vi "Read Tuner Type.vi"(8 "error in (no error)":errorcluster, 11 "RTL-SDR in":refnum<class "Session.lvclass">) -> (0 "error out":errorcluster, 3 "RTL-SDR out":refnum<class "Session.lvclass">)   [LabVIEW 2020, in "RTL-SDR.lvlib" / "Session.lvclass"]
uses:
  Session.lvclass
  Tuner Type.ctl
  RTL-SDR.lvlib
  C:/dev/IlluminatedG/lv-rtl-sdr/lib/librtlsdr.dll
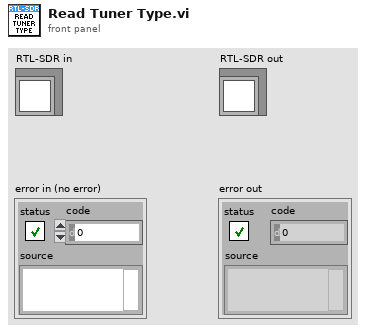
[diagram p1: front panel]
types:
  T1 = typedef "RTL-SDR.lvlib/Tuner Type.ctl" = enum32{"Unknown", "E4000", "FC0012", "FC0013", "FC2580", "R820T", "R828D"}
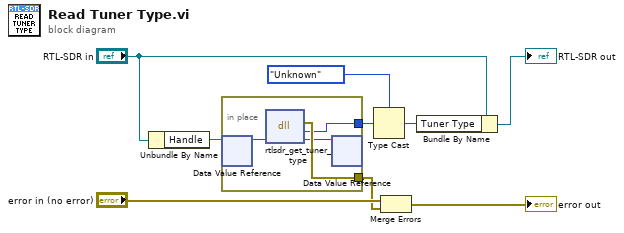
[diagram p0: block diagram]
diagram:
  n1 = Unbundle By Name("RTL-SDR in") -> ("Handle"=w1:refnum<data-value>)
  n2 = in-place {
    in-place-border: [w13] -> w6
    in-place-border: [w12] -> w5
    n3 = in-place-dvr #1(w1) -> (w11:u64)  [unwired: 1 out]
    n4 = dll-call lib="C:/dev/IlluminatedG/lv-rtl-sdr/lib/librtlsdr.dll" fn="rtlsdr_get_tuner_type"("dev"=w11) -> (error out=w13:errorcluster, "return type"=w12:i32, "dev"=w10:u64)  [unwired: 3 in, 1 out]
    n5 = in-place-dvr #1(w10) -> ()  [unwired: 2 out]
  }
  n6 = Type Cast(type=Tuner_Type."Unknown" ("Tuner Type"), x=w5) -> (*(type *) &x=w3:T1)
  n7 = Merge Errors("error in (no error)", w6) -> (→"error out":errorcluster)
  n8 = Bundle By Name(cluster="RTL-SDR in", "Tuner Type"=w3) -> (→"RTL-SDR out":refnum<class "Session.lvclass">)
